vi "Init Definitions.vi"(8 "error in (no error)":errorcluster) -> (0 "error out (no error)":errorcluster)   [LabVIEW 2020, in "JSON Schema Generator.lvlib"]
uses:
  JSON Schema Generator.lvlib
  Defintion FGV Actions.ctl
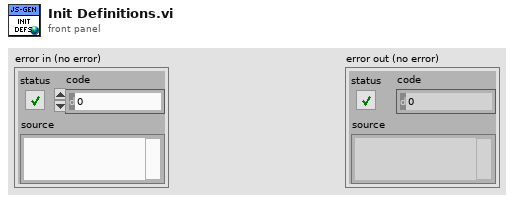
[diagram p1: front panel]
types:
  T1 = typedef "JSON Schema Generator.lvlib/Defintion FGV Actions.ctl" = enum16{"Create Defs", "Update Defs", "Get all Defs", "Get Def"}
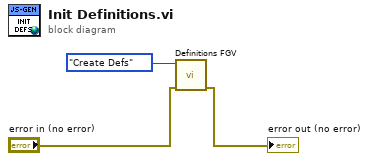
[diagram p0: block diagram]
diagram:
  n1 = call "Definitions FGV.vi"("error in (no error)"="error in (no error)", "Action"=Defintion_FGV_Actions."Create Defs") -> ("error out"=→"error out (no error)":errorcluster)  [unwired: 7 in, 2 out]
